vi "DuplicateHawkeyeConfig.vi"(8 "error in (no error)":errorcluster, 11 "Repo / Workspace Folder Path":path) -> (0 "error out":errorcluster)   [LabVIEW 2019, in "Hawkeye.lvlib"]
uses:
  Hawkeye.lvlib
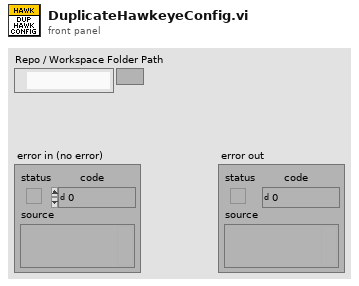
[diagram p1: front panel]
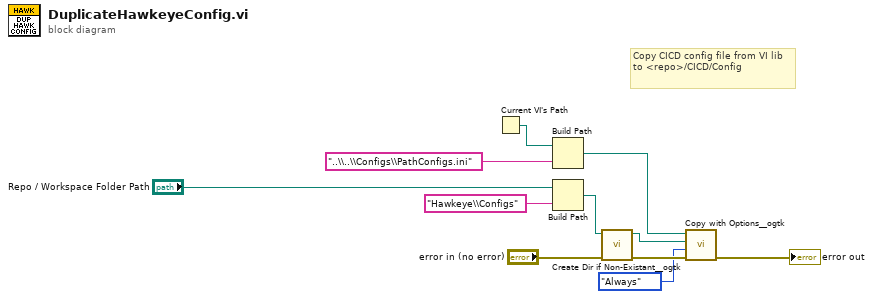
[diagram p0: block diagram]
diagram:
  # "Copy CICD config file from VI lib to <repo>/CICD/Config"
  n1 = Current VI's Path() -> (path=w4:path)
  n2 = Build Path(base path=w4, name or relative path="..\\..\\Configs\\PathConfigs.ini") -> (appended path=w7:path)
  n3 = Build Path(base path="Repo / Workspace Folder Path", name or relative path="Hawkeye\\Configs") -> (appended path=w9:path)
  n4 = call <userlib>:"Create Dir if Non-Existant__ogtk.vi"("error in (no error)"="error in (no error)", "Directory Path"=w9) -> ("error out"=w6:errorcluster, "dup Directory Path"=w8:path)  [unwired: 7 in, 1 out]
  n5 = call <userlib>:"Copy with Options__ogtk.vi"("error in (no error)"=w6, "Replace Mode (Never)"=enum16{"Never", "Always", "If Newer"}."Always", "target path"=w8, "source path"=w7) -> ("error out"=→"error out":errorcluster)  [unwired: 6 in, 1 out]
